vi "_word.GetTableInBookmark.vi"(7 "bookmark (Word)":string, 8 "error in (no error)":errorcluster, 11 "word.document":refnum<k7>) -> (0 "error out":errorcluster, 1 "bookmark to existing table?":bool, 2 "table ref":refnum<k7>, 3 "Tables":refnum<k7>)   [LabVIEW 2018, in "WordReportGeneration.lvlib"]
uses:
  WordReportGeneration.lvlib
  <vilib>/Utility/NIReport.llb/NI_ReportGenerationCore.lvlib
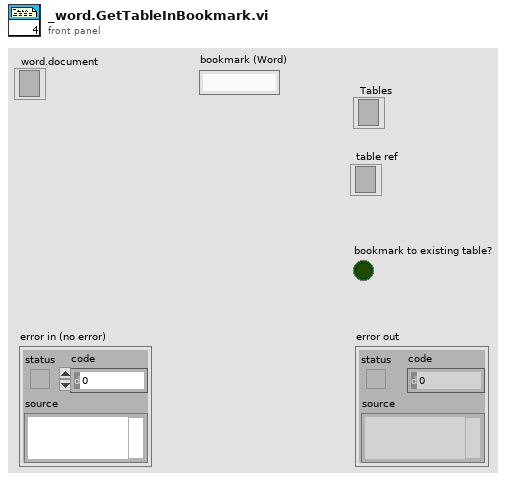
[diagram p1: front panel]
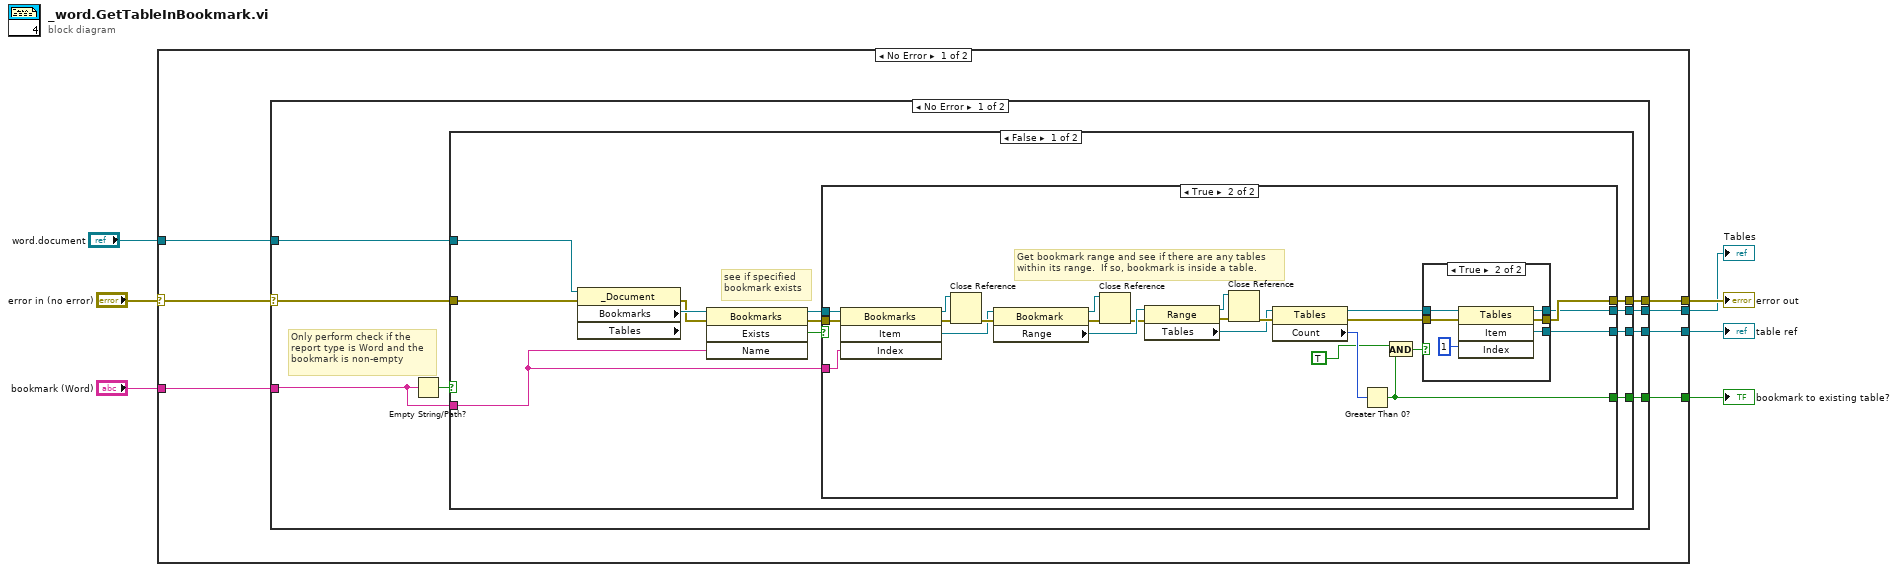
[diagram p0: block diagram]
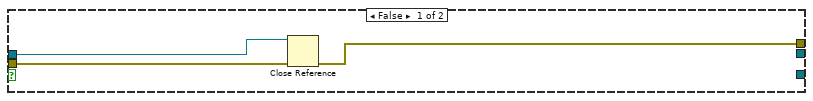
[diagram p2: hidden frame]
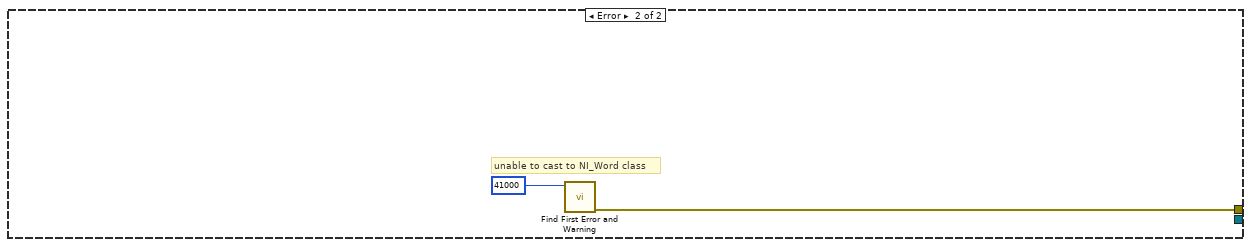
[diagram p5: hidden frame]
diagram:
  n1 = case shown="No Error" "error in (no error)" {
    selector: "error in (no error)" -> [w10 w73]
    tunnel: [w13 w73] -> w6
    tunnel: "bookmark (Word)" -> [w14 _]
    tunnel: [w12 _] -> w4
    tunnel: [w11 _] -> w3
    tunnel: "word.document" -> [w9 _]
    tunnel: [w8 _] -> w1
    frame No Error {
      n2 = case shown="No Error" w10 {
        selector: w10 -> [w18 _]
        tunnel: w14 -> [w16 _]
        tunnel: [w21 w71] -> w13
        tunnel: [w20 _] -> w12
        tunnel: [w19 _] -> w11
        tunnel: w9 -> [w17 _]
        tunnel: [w15 _] -> w8
        frame No Error {
          # "Only perform check if the\nreport type is Word and the\nbookmark is non-empty"
          n3 = Empty String/Path?(string/path=w16) -> (empty?=w22:bool)
          n4 = case shown="False" w22 {
            tunnel: w18 -> [w25 w70]
            tunnel: [w28 w70] -> w21
            tunnel: [w31 _] -> w19
            tunnel: w16 -> [w29 _]
            tunnel: [w26 _] -> w20
            tunnel: w17 -> [w24 _]
            tunnel: [w23 _] -> w15
            frame False {
              # "see if specified\nbookmark exists"
              n5 = property class="_Document" props=["Bookmarks", "Tables"](reference=w24, error in=w25) -> (error out=w27:errorcluster, "Bookmarks"=w34:refnum<k7>)  [unwired: 2 out]
              n6 = invoke class="Bookmarks" method="Exists"(reference=w34, error in=w27, "Name"=w29) -> (reference out=w30:refnum<k7>, error out=w33:errorcluster, "Exists"=w32:bool)  [unwired: 1 in, 1 out]
              n7 = case shown="True" w32 {
                tunnel: w33 -> [w37 w59]
                tunnel: [_ w41] -> w31
                tunnel: w30 -> [w36 w61]
                tunnel: w29 -> [_ w60]
                tunnel: [w35 w39] -> w28
                tunnel: [_ w43] -> w26
                tunnel: [_ w38] -> w23
                frame False {
                  n8 = Close Reference(reference=w36, error in (no error)=w37) -> (error out=w35:errorcluster)
                }
                frame True {
                  # "Get bookmark range and see if there are any tables\nwithin its range.  If so, bookmark is inside a table."
                  n9 = invoke class="Bookmarks" method="Item"(reference=w61, error in=w59, "Index"=w60) -> (reference out=w57:refnum<k7>, error out=w58:errorcluster, "Item"=w55:refnum<k7>)  [unwired: 1 in, 1 out]
                  n10 = Close Reference(reference=w57, error in (no error)=w58) -> (error out=w56:errorcluster)
                  n11 = property class="Bookmark"(reference=w55, error in=w56) -> (reference out=w53:refnum<k7>, error out=w54:errorcluster, "Range"=w52:refnum<k7>)
                  n12 = Close Reference(reference=w53, error in (no error)=w54) -> (error out=w51:errorcluster)
                  n13 = property class="Range"(reference=w52, error in=w51) -> (reference out=w49:refnum<k7>, error out=w50:errorcluster, "Tables"=w46:refnum<k7>)
                  n14 = Close Reference(reference=w49, error in (no error)=w50) -> (error out=w48:errorcluster)
                  n15 = property class="Tables"(reference=w46, error in=w48) -> (reference out=w44:refnum<k7>, error out=w45:errorcluster, "Count"=w47:i32)
                  n16 = Greater Than 0?(x=w47) -> (x > 0?=w41:bool)
                  n17 = And(x=TRUE ("get table ref?"), y=w41) -> (x .and. y?=w42:bool)
                  n18 = case shown="True" w42 {
                    tunnel: w45 -> [w63 w69]
                    tunnel: w44 -> [w62 w68]
                    tunnel: [w63 w67] -> w39
                    tunnel: [w62 w66] -> w38
                    tunnel: [_ w65] -> w43
                    frame False {
                    }
                    frame True {
                      n19 = invoke class="Tables" method="Item"(reference=w68, error in=w69, "Index"=1) -> (reference out=w66:refnum<k7>, error out=w67:errorcluster, "Item"=w65:refnum<k7>)  [unwired: 1 in, 1 out]
                    }
                  }
                }
              }
            }
            frame True {
            }
          }
        }
        frame Error {
          # "unable to cast to NI_Word class"
          n20 = call <vilib>:"Find First Error and Warning.vi"("error code"=41000) -> ("error out"=w71:errorcluster)  [unwired: 2 in, 4 out]
        }
      }
    }
    frame Error {
    }
  }
  "error out" <- w6
  "bookmark to existing table?" <- w3
  "table ref" <- w4
  "Tables" <- w1
